vi "VIPM_build_trial.vi"() -> ()   [LabVIEW 2020]
uses:
  <vilib>/JKI/VIPM API/VIPM API_vipm_api.lvlib
panel:
  in  "Error in":errorcluster
  in  "Build Spec I/P":path=path "C:/Users/sadhana.suresh/Documents/GIT/YouTube_Trial/LabviewJenkinsExample/.vipb"
  out "Build Output":path
  out "Error out":errorcluster
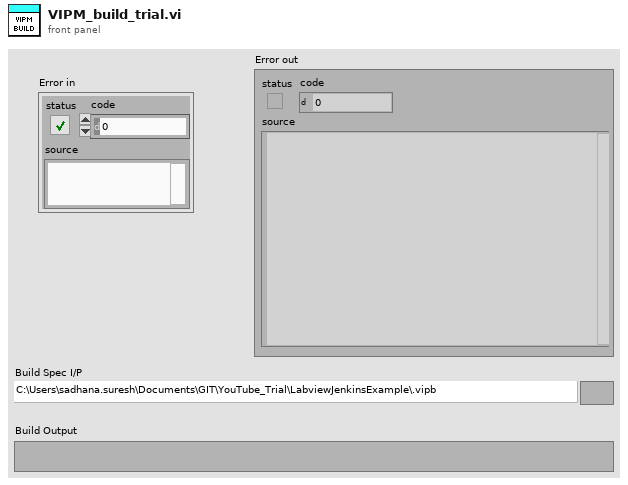
[diagram p1: front panel]
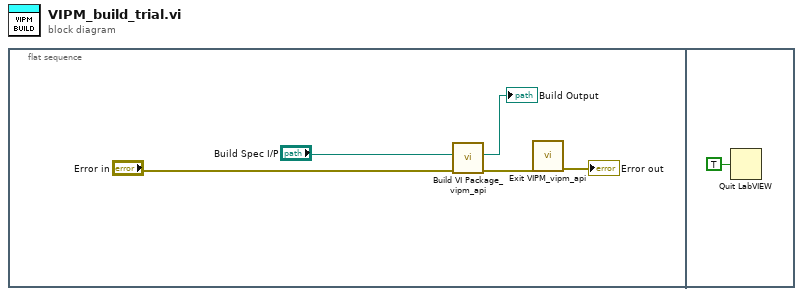
[diagram p0: block diagram]
diagram:
  n1 = flat-sequence {
    frame #0 {
      n2 = call <vilib>:"Build VI Package_vipm_api.vi"("error in (no error)"="Error in", "Path to VIPB File"="Build Spec I/P") -> ("error out"=w5:errorcluster, "Build Output"=→"Build Output":path)  [unwired: 8 in]
      n3 = call <vilib>:"Exit VIPM_vipm_api.vi"("error in (no error)"=w5) -> ("error out"=→"Error out":errorcluster)  [unwired: 10 in]
    }
    frame #1 {
      n4 = Quit LabVIEW(quit? (T)=TRUE) -> ()
    }
  }
